vi "Billard2025.vi"(5 "Open PDF":bool, 7 "balll size":i32=13, 8 "band touch win":u32(colorbox)=6618880, 9 "band touch loose":u32(colorbox)=16711680, 10 "Create matlab score sheet":bool, 11 "path":path) -> (0 "error out":errorcluster, 1 "?":string)   [LabVIEW 2025]
doc: "Le VI principal parcourt les images PNG de la séquence, détecte d’abord la zone du billard (cadre bleu foncé) avec FindBillardBox, puis pour chaque frame calcule la position des 3 boules avec FrameToPosition (création de Pixmap.bin, exécution de Pix2Pos, lecture de Pos.txt).\nSi l’option Create Matlab score sheet est activée, il génère et lance MATLAB (via MatlabScript puis RunMatlab) pour produire le ScoreSheet…pdf et le Summary…txt, et peut ouvrir automatiquement le PDF selon le bouton Open PDF"
panel:
  in  "Dark Blue Frame":T1={"Rmin"=0.0, " Rmax"=24.0, "Gmin"=0.0, "Gmax"=49.0, "Bmin"=100.0, "Bmax"=119.0}
  # "summary"
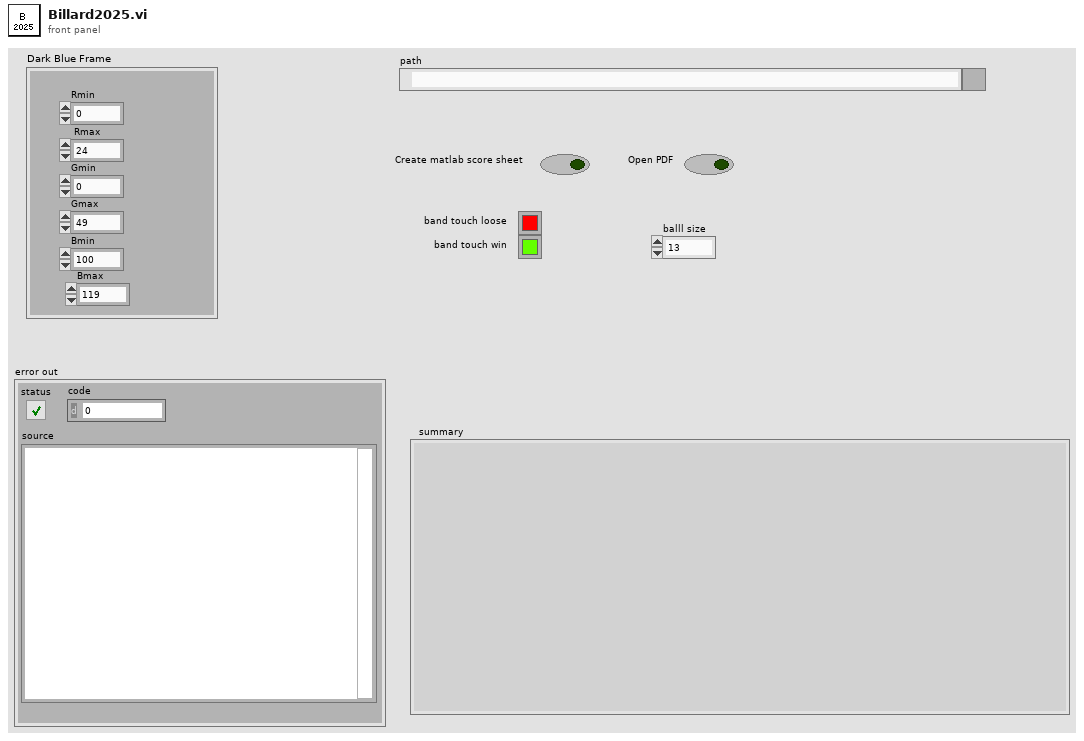
[diagram p1: front panel]
types:
  T1 = cluster{"Rmin":dbl, " Rmax":dbl, "Gmin":dbl, "Gmax":dbl, "Bmin":dbl, "Bmax":dbl}
  T2 = cluster{"Xmin":dbl, "Xmax":dbl, "Ymin":dbl, "Ymax":dbl}
  T3 = enum16{"open", "replace", "create", "open or create", "replace or create", "replace or create with confirmation"}
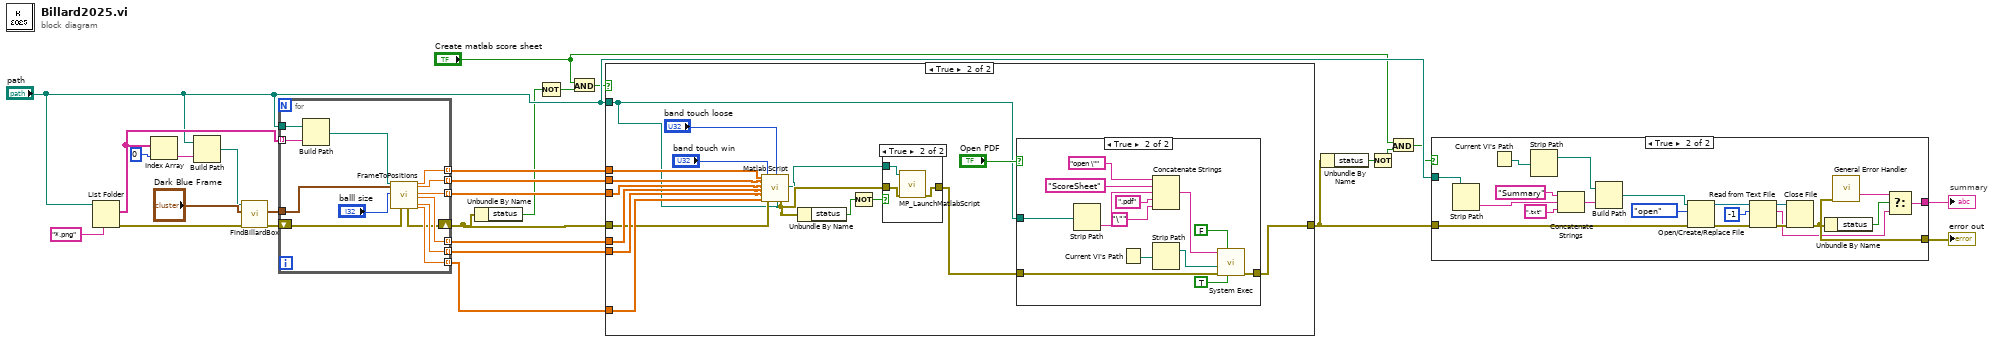
[diagram p0: block diagram]
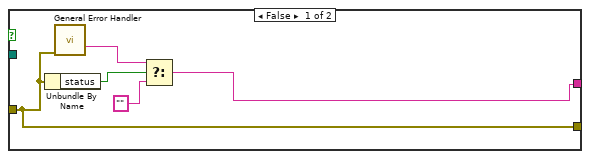
[diagram p5: hidden frame]
diagram:
  # "summary"
  n1 = List Folder(path="path", pattern="*.png") -> (filenames=w19:string[], error out=w23:errorcluster)  [unwired: 2 in, 2 out]
  n2 = Index Array(array=w19, index=0) -> (element=w18:string)
  n3 = Build Path(base path="path", name or relative path=w18) -> (appended path=w17:path)
  n4 = call "FindBillardBox.vi"("error in (no error)"=w23, "Dark Blue Frame"="Dark Blue Frame", "Path"=w17) -> ("error out"=w25:errorcluster, "Billard Box"=w24:T2)  [unwired: 7 in]
  n5 = for {
    tunnel: "path" -> [w40]
    tunnel: w24 -> [w39]
    tunnel: [w37] -> w15 mode=indexing
    tunnel: [w36] -> w14 mode=indexing
    tunnel: [w35] -> w13 mode=indexing
    tunnel: [w34] -> w12 mode=indexing
    tunnel: [w33] -> w11 mode=indexing
    tunnel: [w32] -> w10 mode=indexing
    tunnel: w19 -> [w30] mode=indexing
    shift-right: [w29] -> w7
    shift-left: w25 -> [w31]
    n6 = Build Path(base path=w40, name or relative path=w30) -> (appended path=w38:path)
    n7 = call "FrameToPositions.vi"("PNG Path"=w38, "Billardbox"=w39, "BallDiameter"="balll size", "error in (no error)"=w31) -> ("error out"=w29:errorcluster, "X red"=w37:dbl, "Y red"=w36:dbl, "X  yellow"=w35:dbl, "Y  yellow"=w34:dbl, "X  white"=w33:dbl, "Y   white"=w32:dbl)  [unwired: 13 in, 4 out]
  }
  n8 = Unbundle By Name(w7) -> ("status"=w8:bool)
  n9 = Not(x=w8) -> (.not. x?=w6:bool)
  n10 = And(x="Create matlab score sheet", y=w6) -> (x .and. y?=w5:bool)
  n11 = case shown="True" w5 {
    tunnel: [w41 w54] -> w16
    tunnel: w15 -> [_ w51]
    tunnel: w14 -> [_ w50]
    tunnel: w13 -> [_ w49]
    tunnel: w12 -> [_ w48]
    tunnel: w11 -> [_ w47]
    tunnel: w10 -> [_ w46]
    tunnel: w7 -> [w41 w45]
    tunnel: "path" -> [_ w44]
    frame False {
    }
    frame True {
      n12 = call "Matlab Script.vi"("Xr"=w51, "Yr"=w50, "Xy"=w49, "Yy"=w48, "Xw"=w47, "Yw"=w46, "Couleur Win"="band touch win", "Error In"=w45, "Couleur Lose"="band touch loose", "Path"=w44) -> ("Error Out"=w43:errorcluster, "Script Path 2"=w42:path)  [unwired: 8 in]
      n13 = Unbundle By Name(w43) -> ("status"=w58:bool)
      n14 = Not(x=w58) -> (.not. x?=w57:bool)
      n15 = case shown="True" w57 {
        tunnel: w42 -> [_ w76]
        tunnel: [w73 w74] -> w55
        tunnel: w43 -> [w73 w75]
        frame False {
        }
        frame True {
          n16 = call "MP_LaunchMatlabScript.vi"("error in (no error)"=w75, "matlab script path"=w76) -> ("error out"=w74:errorcluster)  [unwired: 4 in, 5 out]
        }
      }
      n17 = case shown="True" "Open PDF" {
        tunnel: w44 -> [_ w62]
        tunnel: [w59 w64] -> w54
        tunnel: w55 -> [w59 w63]
        frame False {
        }
        frame True {
          n18 = Strip Path(path=w62) -> (name=w71:string)  [unwired: 1 out]
          n19 = Current VI's Path() -> (path=w60:path)
          n20 = Concatenate Strings("open \"" ("string"), "ScoreSheet" ("string"), w71, ".pdf" ("string"), "\"" ("string")) -> (w68:string)
          n21 = Strip Path(path=w60) -> (stripped path=w61:path)  [unwired: 1 out]
          n22 = call <vilib>:"System Exec.vi"("run minimized? (F)"=TRUE, "wait until completion? (T)"=FALSE, "error in (no error)"=w63, "working directory"=w61, "command line"=w68) -> ("error out"=w64:errorcluster)  [unwired: 3 in, 3 out]
        }
      }
    }
  }
  n23 = Unbundle By Name(w16) -> ("status"=w4:bool)
  n24 = Not(x=w4) -> (.not. x?=w3:bool)
  n25 = And(x="Create matlab score sheet", y=w3) -> (x .and. y?=w2:bool)
  n26 = case shown="True" w2 {
    tunnel: w16 -> [w79 w96]
    tunnel: [w79 w86] -> w27
    tunnel: "path" -> [_ w91]
    tunnel: [w78 w84] -> w26
    frame False {
      n27 = Unbundle By Name(w79) -> ("status"=w81:bool)
      n28 = call <vilib>:"General Error Handler.vi"("error in (no error)"=w79) -> ("message"=w80:string)  [unwired: 10 in, 4 out]
      n29 = Select(t=w80, s=w81, f="") -> (s? t:f=w78:string)
    }
    frame True {
      n30 = Strip Path(path=w91) -> (name=w92:string)  [unwired: 1 out]
      n31 = Current VI's Path() -> (path=w83:path)
      n32 = Strip Path(path=w83) -> (stripped path=w82:path)  [unwired: 1 out]
      n33 = Concatenate Strings("Summary" ("string"), w92, ".txt" ("string")) -> (w89:string)
      n34 = Build Path(base path=w82, name or relative path=w89) -> (appended path=w100:path)
      n35 = Open/Create/Replace File(file path (use dialog)=w100, error in=w96, operation (0:open)=T3."open") -> (refnum out=w99:refnum<file>, error out=w95:errorcluster)  [unwired: 3 in, 1 out]
      n36 = Read from Text File(file (use dialog)=w99, count=-1, error in=w95) -> (refnum out=w98:refnum<file>, text=w85:string, error out=w97:errorcluster)  [unwired: 1 in, 1 out]
      n37 = Close File(refnum=w98, error in=w97) -> (error out=w86:errorcluster)  [unwired: 1 out]
      n38 = Unbundle By Name(w86) -> ("status"=w88:bool)
      n39 = call <vilib>:"General Error Handler.vi"("error in (no error)"=w86) -> ("message"=w87:string)  [unwired: 10 in, 4 out]
      n40 = Select(t=w87, s=w88, f=w85) -> (s? t:f=w84:string)
    }
  }
  "?" <- w26
  "error out" <- w27
